vi "add length to message.vi"(10 "header byte":string, 11 "message":string) -> (3 "message out":string)   [LabVIEW 2019, in "PG_LIB.lvlib" / "Postgres Connector.lvclass"]
uses:
  Postgres Connector.lvclass
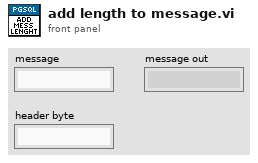
[diagram p1: front panel]
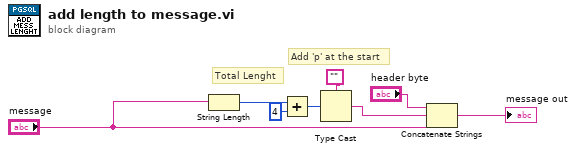
[diagram p0: block diagram]
diagram:
  # "Total Lenght"
  # "Add 'p' at the start"
  n1 = String Length(string="message") -> (length=w2:i32)
  n2 = Add(x=w2, y=4) -> (x+y=w4:i32)
  n3 = Type Cast(type="", x=w4) -> (*(type *) &x=w1:string)
  n4 = Concatenate Strings("header byte", w1, "message") -> (→"message out":string)
